vi "displayHoloListEnum.vi"(8 "error in (no error)":errorcluster, 10 "path":path[](array[path]), 11 "Ring in":refnum<vi>) -> (0 "error out":errorcluster)   [LabVIEW 2023]
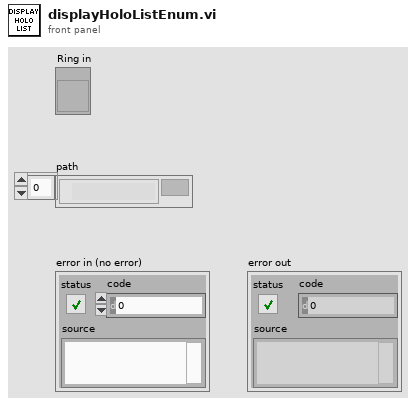
[diagram p1: front panel]
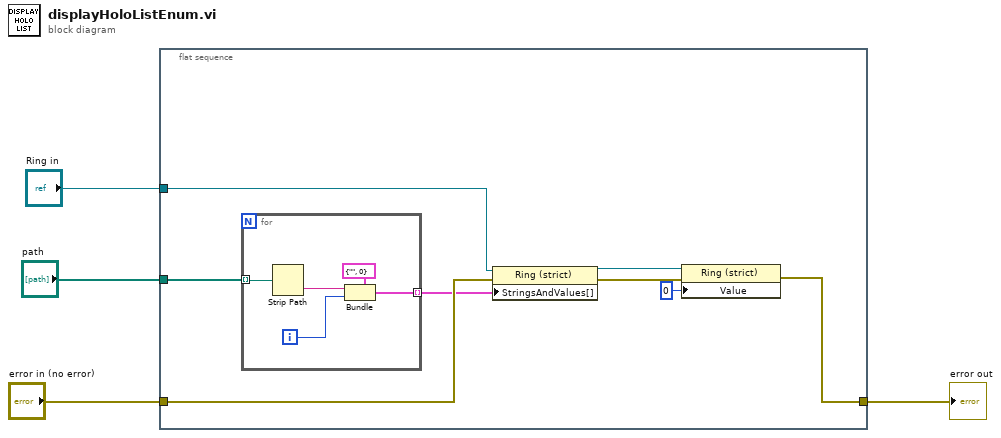
[diagram p0: block diagram]
diagram:
  n1 = flat-sequence {
    tunnel: "Ring in" -> [w11]
    tunnel: "error in (no error)" -> [w10]
    tunnel: [w6] -> w3
    tunnel: "path" -> [w12]
    frame #0 {
      n2 = for {
        tunnel: w12 -> [w17] mode=indexing
        tunnel: [w13] -> w9 mode=indexing
        i -> [w14]
        n3 = Strip Path(path=w17) -> (name=w15:string)  [unwired: 1 out]
        n4 = Bundle(cluster=cluster{"String":string, "Value":u16} {"String"="", "Value"=0}, "String"=w15, "Value"=w14) -> (w13:cluster{"String":string, "Value":u16})
      }
      n5 = property class="Ring (strict)"(reference=w11, error in=w10, "StringsAndValues[]"=w9) -> (reference out=w8:refnum<vi>, error out=w7:errorcluster)
      n6 = property class="Ring (strict)"(reference=w8, error in=w7, "Value"=u16 0) -> (error out=w6:errorcluster)  [unwired: 1 out]
    }
  }
  "error out" <- w3
